vi "_Destroy.vi"(8 "error in (no error)":errorcluster, 11 "Scanner in":refnum<class "Scanner.lvclass">) -> (0 "error out":errorcluster, 2 "finalized Scannable":refnum<class "Scannable.lvclass">)   [LabVIEW 2009, in "Scanner.lvclass"]
doc: "Release resources from and deallocate this Scanner instance."
uses:
  Scanner.lvclass
  Instruments/Utility Classes/Scannable/Scannable.lvclass
  Scanner.lvclass/Scanner.ctl
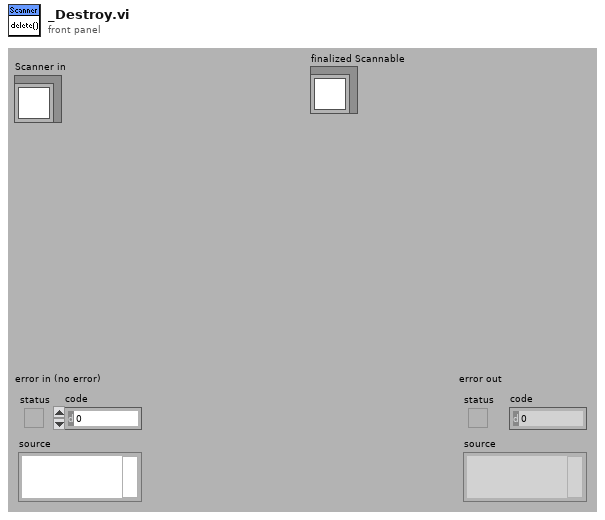
[diagram p1: front panel]
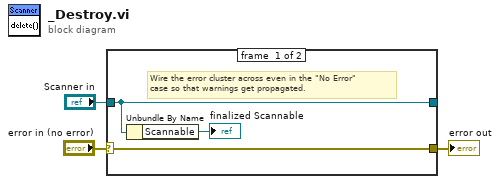
[diagram p0: block diagram]
diagram:
  n1 = case shown="No Error" "error in (no error)" {
    selector: "error in (no error)" -> [w6 w8]
    tunnel: [w6 w8] -> w2
    tunnel: [w5 w7] -> _
    tunnel: "Scanner in" -> [w5 w7]
    frame #0 {
      # "Wire the error cluster across even in the \"No Error\"\ncase so that warnings get propagated."
      n2 = Unbundle By Name(w5) -> ("Scannable"=→"finalized Scannable":refnum<class "Scannable.lvclass">)
    }
    frame #1 {
    }
  }
  "error out" <- w2
